vi "Head and Tail Detection Angle Based (SubVI).vi"(0 "Boundary Point XY":u32, 1 "Bondary Valid?":bool, 2 "Scan End?":bool) -> (9 "Mean Angle":fxp<+/-,32,16> format="%.21g", 11 "Ready for Input?":bool, 14 "Output Valid?":bool, 15 "Skip Contour Analysis":bool, 16 "Significant Angle Diff?":bool, 17 "V1 (ID)":u16, 18 "V2 (ID)":u16, 19 "N Points":u16)   [LabVIEW 2015]
uses:
  Controls (FPGA)/Find Peak Angle.ctl
  <vilib>/rvi/Emulation/niFpgaSctlEmulationGetInTimedLoop.vi
  <vilib>/rvi/Emulation/niFpgaProcessEmulError.vi
  <vilib>/rvi/Memory/Memory_Emulation/nirvimemoryFastEmulation.vi
  <vilib>/rvi/Memory/Memory_Emulation/nirvimemoryEmulation.vi
  <vilib>/rvi/Emulation/niFpgaEmulationIsFPGAContextNoSignature.vi
  <vilib>/rvi/DataTransferAndStorage/Container/Common/niFpgaContainerGetUniqueNameForEmu.vi
  <vilib>/rvi/errors/nirviReportUnexpectedCaseInternalError (U32).vi
  <vilib>/rvi/DataTransferAndStorage/Container/XNode/niFpgaContainer.xnode
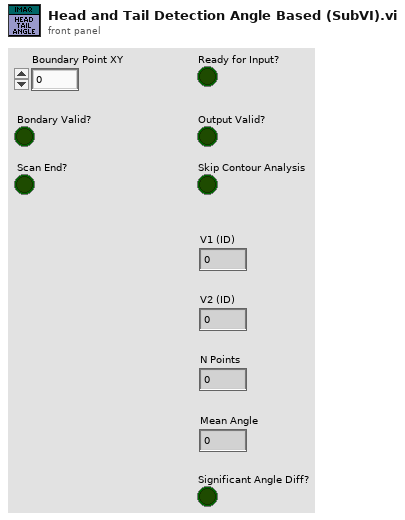
[diagram p1: front panel]
types:
  T1 = typedef "Find Peak Angle.ctl" = enum16{"Wait", "Find Peak"}
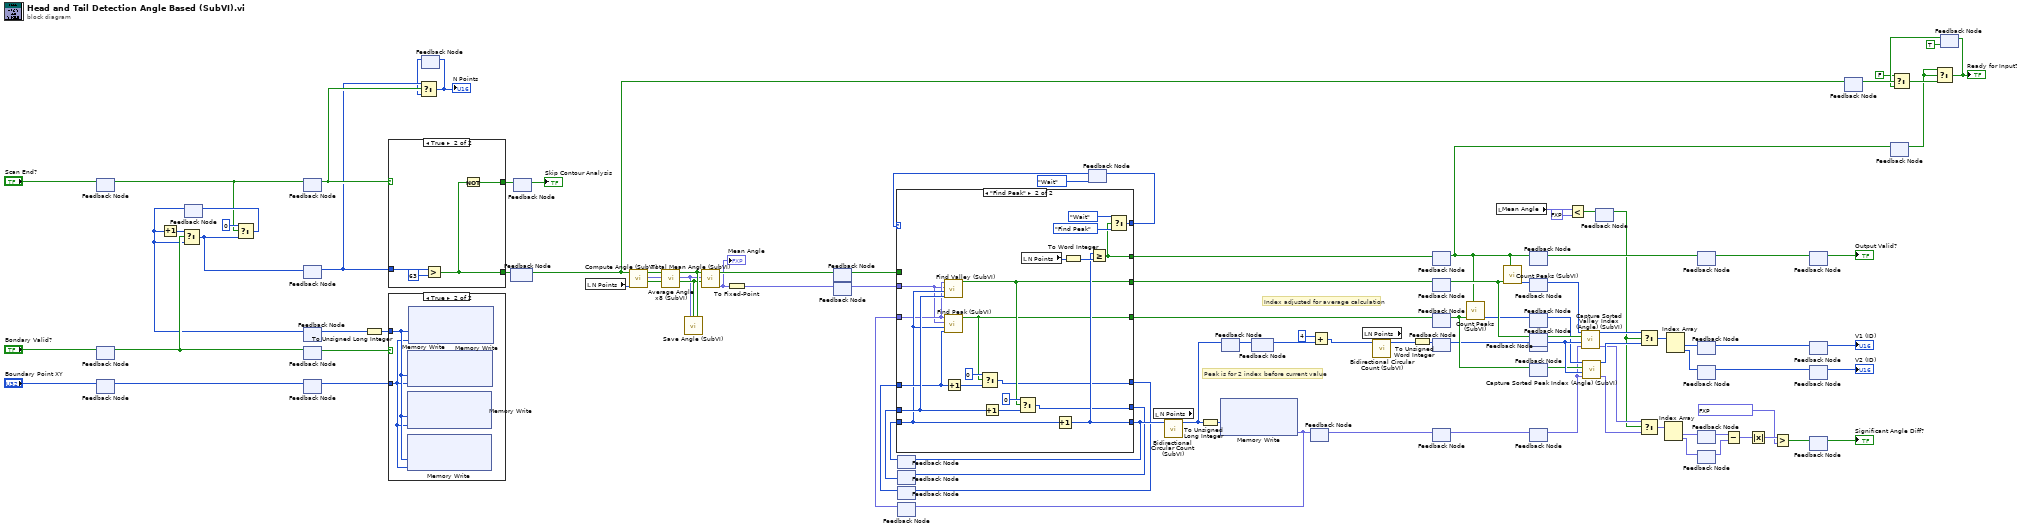
[diagram p0: block diagram]
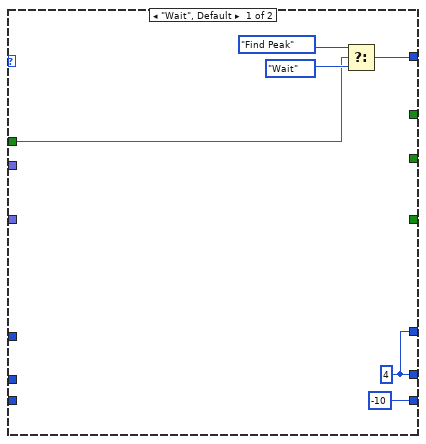
[diagram p2: hidden frame]
diagram:
  # "Index adjusted for average calculation"
  # "Peak is for 2 index before current value"
  n1 = feedback-in #1("Scan End?") -> ()
  n2 = feedback #1() -> (w76:bool)  [unwired: 1 in]
  n3 = feedback-in #2("Bondary Valid?") -> ()
  n4 = feedback #2() -> (w75:bool)  [unwired: 1 in]
  n5 = feedback-in #3("Boundary Point XY") -> ()
  n6 = feedback #3() -> (w105:u32)  [unwired: 1 in]
  n7 = feedback #4() -> (w45:u16)  [unwired: 1 in]
  n8 = Increment(x=w45) -> (x+1=w46:u16)
  n9 = Select(t=w46, s=w75, f=w45) -> (s? t:f=w74:u16)
  n10 = Select(t=u16 0 ("Count"), s=w76, f=w74) -> (s? t:f=w77:u16)
  n11 = feedback-in #4(w77) -> ()
  n12 = feedback-in #5(w76) -> ()
  n13 = feedback #5() -> (w70:bool)  [unwired: 1 in]
  n14 = feedback-in #6(w74) -> ()
  n15 = feedback #6() -> (w69:u16)  [unwired: 1 in]
  n16 = feedback-in #7(w45) -> ()
  n17 = feedback #7() -> (w73:u16)  [unwired: 1 in]
  n18 = feedback-in #8(w75) -> ()
  n19 = feedback #8() -> (w71:bool)  [unwired: 1 in]
  n20 = feedback-in #9(w105) -> ()
  n21 = feedback #9() -> (w72:u32)  [unwired: 1 in]
  n22 = To Unsigned Long Integer(number=w73) -> (unsigned 32bit integer=w104:u32)
  n23 = case shown="True" w71 {
    tunnel: w72 -> [_ w109]
    tunnel: w104 -> [_ w110]
    frame False {
    }
    frame True {
      n24 = xnode ("Memory Write")("Address"=w110, "Data"=w109) -> ()  [unwired: 1 in, 1 out]
      n25 = xnode ("Memory Write")("Address"=w110, "Data"=w109) -> ()  [unwired: 1 in, 1 out]
      n26 = xnode ("Memory Write")("Address"=w110, "Data"=w109) -> ()  [unwired: 1 in, 1 out]
      n27 = xnode ("Memory Write")("Address"=w110, "Data"=w109) -> ()  [unwired: 1 in, 1 out]
    }
  }
  n28 = case shown="True" w70 {
    tunnel: w69 -> [_ w114]
    tunnel: [_ w112] -> w103
    tunnel: [_ w111] -> w102
    frame False {
    }
    frame True {
      n29 = Greater?(x=w114, y=u16 63) -> (0:w112:bool)
      n30 = Not(x=w112) -> (.not. x?=w111:bool)
    }
  }
  n31 = feedback #10() -> (w68:u16)  [unwired: 1 in]
  n32 = Select(t=w69, s=w70, f=w68) -> (s? t:f=w67:u16)
  "N Points" <- w67
  n33 = feedback-in #10(w67) -> ()
  n34 = feedback-in #11(w103) -> ()
  n35 = feedback #11() -> (w65:bool)  [unwired: 1 in]
  n36 = feedback-in #12(w102) -> ()
  n37 = feedback #12() -> (→"Skip Contour Analysis":bool)  [unwired: 1 in]
  n38 = local read "N Points"() -> (w66:u16)
  n39 = call "Compute Angle (SubVI).vi"("N Points"=w66, "Start"=w65) -> ("Angle Valid?"=w42:bool, "Angle"=w43:fxp<+/-,16,3>, "Done?"=w44:bool)  [unwired: 7 in]
  n40 = call "Average Angle x8 (SubVI).vi"("In Valid?"=w42, "Angle In"=w43, "End?"=w44) -> ("Out Valid?"=w29:bool, "Angle Out"=w28:fxp<+/-,16,3>, "Done?"=w40:bool)  [unwired: 6 in]
  n41 = call "Save Angle (SubVI).vi"("Angle"=w28, "In Valid?"=w29, "Done?"=w40) -> ()  [unwired: 13 in]
  n42 = call "Total Mean Angle (SubVI).vi"("Angle Valid"=w29, "Angle"=w28, "Done In"=w40) -> ("Mean Angle"=w25:fxp<+/-,32,16>, "Done Out"=w41:bool)  [unwired: 7 in]
  "Mean Angle" <- w25
  n43 = To Fixed-Point(number=w25) -> (fixed-point=w24:fxp<+/-,16,3>)  [unwired: 1 in]
  n44 = feedback-in #13(w41) -> ()
  n45 = feedback #13() -> (w64:bool)  [unwired: 1 in]
  n46 = feedback-in #14(w24) -> ()
  n47 = feedback #14() -> (w63:fxp<+/-,16,3>)  [unwired: 1 in]
  n48 = feedback #15() -> (w84:i16)  [unwired: 1 in]
  n49 = feedback #16() -> (w58:u16)  [unwired: 1 in]
  n50 = feedback #17() -> (w56:u16)  [unwired: 1 in]
  n51 = feedback #18() -> (w100:fxp<+/-,16,3>)  [unwired: 1 in]
  n52 = feedback #19(Find_Peak_Angle."Wait") -> (w98:T1)
  n53 = case shown="\"Find Peak\"" w98 {
    tunnel: [w120 w140] -> w99
    tunnel: w100 -> [_ w122]
    tunnel: [_ w136] -> w96
    tunnel: w64 -> [w117 _]
    tunnel: [_ w131] -> w26
    tunnel: [i16 -10 ("Count Out") w134] -> w60
    tunnel: w84 -> [_ w123]
    tunnel: w63 -> [_ w121]
    tunnel: [w115 w133] -> w59
    tunnel: w58 -> [_ w130]
    tunnel: [w115 w126] -> w57
    tunnel: w56 -> [_ w125]
    tunnel: [_ w124] -> w27
    frame "Wait", Default {
      w115 = u16 4 ("Count Out")
      n54 = Select(t=Find_Peak_Angle."Find Peak", s=w117, f=Find_Peak_Angle."Wait") -> (s? t:f=w120:T1)
    }
    frame "Find Peak" {
      n55 = call "Find Valley (SubVI).vi"("Last Valley Distance"=w130, "Index"=w123, "Min Angle"=w121, "Angle"=w122) -> ("Valley?"=w131:bool)  [unwired: 7 in]
      n56 = call "Find Peak (SubVI).vi"("Last Peak Distance"=w125, "Index"=w123, "Max Angle"=w121, "Angle"=w122) -> ("Peak?"=w124:bool)  [unwired: 7 in]
      n57 = Increment(x=w125) -> (x+1=w128:u16)
      n58 = Select(t=u16 0, s=w124, f=w128) -> (s? t:f=w126:u16)
      n59 = Increment(x=w130) -> (x+1=w129:u16)
      n60 = Select(t=u16 0, s=w131, f=w129) -> (s? t:f=w133:u16)
      n61 = local read "N Points"() -> (w137:u16)
      n62 = Increment(x=w123) -> (x+1=w134:i16)
      n63 = To Word Integer(number=w137) -> (16bit integer=w135:i16)
      n64 = Greater Or Equal?(x=w134, y=w135) -> (x >= y?=w136:bool)
      n65 = Select(t=Find_Peak_Angle."Wait", s=w136, f=Find_Peak_Angle."Find Peak") -> (s? t:f=w140:T1)
    }
  }
  n66 = feedback-in #15(w60) -> ()
  n67 = feedback-in #16(w59) -> ()
  n68 = feedback-in #17(w57) -> ()
  n69 = feedback-in #19(w99) -> ()
  n70 = local read "N Points"() -> (w62:u16)
  n71 = call "Bidirectional Circular Count (SubVI).vi"("Max. Count"=w62, "Count In"=w60) -> ("Count Out"=w61:i16)  [unwired: 9 in]
  n72 = To Unsigned Long Integer(number=w61) -> (unsigned 32bit integer=w95:u32)
  n73 = xnode ("Memory Write")("Address"=w95) -> ("Data"=w33:fxp<+/-,16,3>)  [unwired: 1 in, 1 out]
  n74 = feedback-in #18(w33) -> ()
  n75 = feedback-in #20(w61) -> ()
  n76 = feedback #20() -> (w85:i16)  [unwired: 1 in]
  n77 = feedback-in #21(w85) -> ()
  n78 = feedback #21() -> (w22:i16)  [unwired: 1 in]
  n79 = feedback #22() -> (w32:fxp<+/-,16,3>)  [unwired: 1 in]
  n80 = feedback-in #22(w33) -> ()
  n81 = Add(x=i16 4, y=w22) -> (x+y=w20:i16)
  n82 = local read "N Points"() -> (w23:u16)
  n83 = call "Bidirectional Circular Count (SubVI).vi"("Max. Count"=w23, "Count In"=w20) -> ("Count Out"=w21:i16)  [unwired: 9 in]
  n84 = To Unsigned Word Integer(number=w21) -> (unsigned 16bit integer=w83:u16)
  n85 = feedback #23() -> (w55:bool)  [unwired: 1 in]
  n86 = feedback-in #23(w96) -> ()
  n87 = feedback #24() -> (w81:bool)  [unwired: 1 in]
  n88 = feedback-in #24(w26) -> ()
  n89 = feedback #25() -> (w54:bool)  [unwired: 1 in]
  n90 = feedback-in #25(w27) -> ()
  n91 = feedback-in #26(w83) -> ()
  n92 = feedback #26() -> (w53:u16)  [unwired: 1 in]
  n93 = feedback #27() -> (w31:fxp<+/-,16,3>)  [unwired: 1 in]
  n94 = feedback-in #27(w32) -> ()
  n95 = call "Count Peaks (SubVI).vi"("Done"=w55, "Increment"=w54) -> ("Peak Count"=w52:u16)  [unwired: 9 in]
  n96 = local read "Mean Angle"() -> (w38:fxp<+/-,32,16>)
  n97 = call "Count Peaks (SubVI).vi"("Done"=w55, "Increment"=w81) -> ("Peak Count"=w82:u16)  [unwired: 9 in]
  n98 = feedback-in #28(w55) -> ()
  n99 = feedback #28() -> (w50:bool)  [unwired: 1 in]
  n100 = feedback-in #29(w82) -> ()
  n101 = feedback #29() -> (w36:u16)  [unwired: 1 in]
  n102 = feedback-in #30(w52) -> ()
  n103 = feedback #30() -> (w35:u16)  [unwired: 1 in]
  n104 = feedback-in #31(w81) -> ()
  n105 = feedback #31() -> (w49:bool)  [unwired: 1 in]
  n106 = feedback-in #32(w53) -> ()
  n107 = feedback #32() -> (w48:u16)  [unwired: 1 in]
  n108 = feedback-in #33(w54) -> ()
  n109 = feedback #33() -> (w47:bool)  [unwired: 1 in]
  n110 = feedback-in #34(w31) -> ()
  n111 = feedback #34() -> (w30:fxp<+/-,16,3>)  [unwired: 1 in]
  n112 = Less?(x=w38, y=fxp<+/-,32,16> 1.0) -> (x < y?=w37:bool)
  n113 = call "Capture Sorted Valley Index (Angle) (SubVI).vi"("Angle"=w30, "Valley Index"=w48, "Dip Valid?"=w49, "Valley Count"=w36) -> ("Anlge Array"=w15:fxp<+/-,16,3>[], "Sorted Valley Index"=w18:u16[])  [unwired: 6 in]
  n114 = call "Capture Sorted Peak Index (Angle) (SubVI).vi"("Angle"=w30, "Peak Index"=w48, "Dip Valid?"=w47, "Peak Count"=w35) -> ("Angle Array"=w14:fxp<+/-,16,3>[], "Sorted Peak Index"=w51:u16[])  [unwired: 6 in]
  n115 = feedback-in #35(w37) -> ()
  n116 = feedback #35() -> (w13:bool)  [unwired: 1 in]
  n117 = Select(t=w18, s=w13, f=w51) -> (s? t:f=w34:u16[])
  n118 = Select(t=w15, s=w13, f=w14) -> (s? t:f=w16:fxp<+/-,16,3>[])
  n119 = Index Array(array=w16) -> (element #1=w12:fxp<+/-,16,3>, element #2=w11:fxp<+/-,16,3>)  [unwired: 2 in]
  n120 = Index Array(array=w34) -> (element #1=w80:u16, element #2=w79:u16)  [unwired: 2 in]
  n121 = feedback-in #36(w50) -> ()
  n122 = feedback #36() -> (w17:bool)  [unwired: 1 in]
  n123 = feedback-in #37(w80) -> ()
  n124 = feedback #37() -> (w87:u16)  [unwired: 1 in]
  n125 = feedback-in #38(w79) -> ()
  n126 = feedback #38() -> (w86:u16)  [unwired: 1 in]
  n127 = feedback #39() -> (w10:fxp<+/-,16,3>)  [unwired: 1 in]
  n128 = feedback-in #39(w12) -> ()
  n129 = feedback #40() -> (w9:fxp<+/-,16,3>)  [unwired: 1 in]
  n130 = feedback-in #40(w11) -> ()
  n131 = Subtract(x=w10, y=w9) -> (x-y=w8:fxp<+/-,17,4>)
  n132 = Absolute Value(x=w8) -> (abs(x)=w7:fxp<+,16,3>)
  n133 = Greater?(x=w7, y=fxp<+,16,3> 0.0999755859375) -> (0:w5:bool)
  n134 = feedback-in #41(w17) -> ()
  n135 = feedback #41() -> (→"Output Valid?":bool)  [unwired: 1 in]
  n136 = feedback-in #42(w87) -> ()
  n137 = feedback #42() -> (→"V1 (ID)":u16)  [unwired: 1 in]
  n138 = feedback-in #43(w86) -> ()
  n139 = feedback #43() -> (→"V2 (ID)":u16)  [unwired: 1 in]
  n140 = feedback-in #44(w5) -> ()
  n141 = feedback #44() -> (→"Significant Angle Diff?":bool)  [unwired: 1 in]
  n142 = feedback #45() -> (w94:bool)  [unwired: 1 in]
  n143 = feedback-in #45(w65) -> ()
  n144 = feedback #46() -> (w89:bool)  [unwired: 1 in]
  n145 = feedback-in #46(w55) -> ()
  n146 = feedback #47(TRUE ("t")) -> (w92:bool)
  n147 = Select(t=FALSE, s=w94, f=w92) -> (s? t:f=w93:bool)
  n148 = Select(t=w89, s=w89, f=w93) -> (s? t:f=w91:bool)
  "Ready for Input?" <- w91
  n149 = feedback-in #47(w91) -> ()
